vi "Input 24 Hour Settings.vi"(7 "GEA2 HyperData":bool=TRUE, 11 "Heating  Mode":T2=enum."Hybrid Heating") -> (4 "GEA2 Set Mode Out":T1=enum."HighDemand", 6 "Set PointOut":u8=140, 8 "GEA2 HyperData Out":bool, 15 "Heating  Mode Out":T2=enum."Hybrid Heating")   [LabVIEW 2014]
uses:
  Utility/GEA2 Commands/HEWH/Type Definitions/HEWH_Mode.ctl
  Type Definitions/Heating Modes.ctl
panel:
  in  "Set Point":u8=135
  in  "Complete":bool
  # "Test Communication Setup"
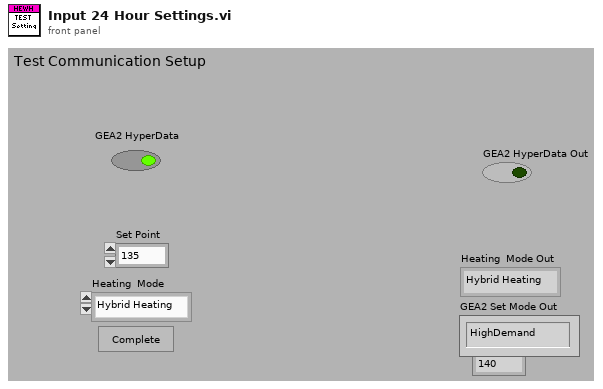
[diagram p1: front panel]
types:
  T1 = typedef "HEWH_Mode.ctl" = enum16{"Hybrid", "Std Electric", "eHeat", "HighDemand", "Vacation"}
  T2 = typedef "Heating Modes.ctl" = enum16{"Standard Electric", "Hybrid Heating", "E-Heat Mode"}
  T3 = typedef "HEWH_Mode.ctl" = enum16{"Hybrid", "StdElectric", "eHeat", "HighDemand", "Vacation"}
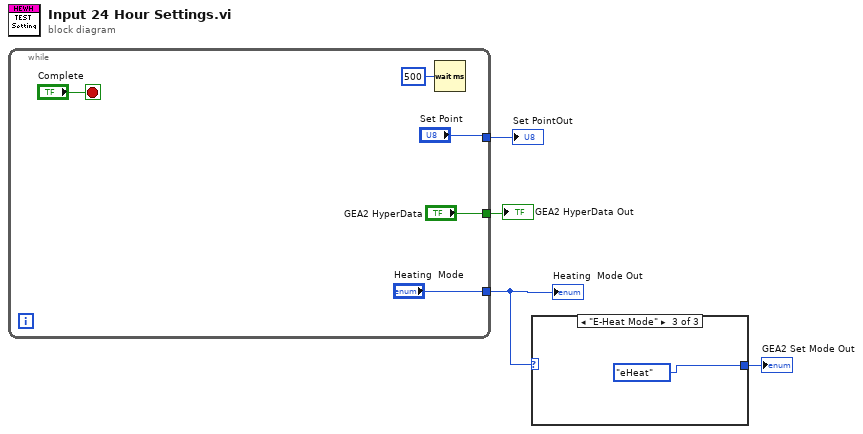
[diagram p0: block diagram]
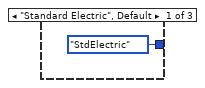
[diagram p2: hidden frame]
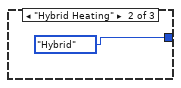
[diagram p3: hidden frame]
diagram:
  n1 = while {
    tunnel: ["GEA2 HyperData"] -> w4
    tunnel: ["Heating  Mode"] -> w2
    tunnel: ["Set Point"] -> w3
    stop <- "Complete" stop-if-true
    n2 = Wait (ms)(milliseconds to wait=u32 500) -> ()  [unwired: 1 out]
  }
  "GEA2 HyperData Out" <- w4
  "Heating  Mode Out" <- w2
  "Set PointOut" <- w3
  n3 = case shown="\"E-Heat Mode\"" w2 {
    tunnel: [HEWH_Mode."StdElectric" ("Mode Out") HEWH_Mode."Hybrid" ("Mode Out") HEWH_Mode."eHeat" ("Mode Out")] -> w1
    frame "Standard Electric", Default {
    }
    frame "Hybrid Heating" {
    }
    frame "E-Heat Mode" {
    }
  }
  "GEA2 Set Mode Out" <- w1
